vi "Connect Websockets.vi"(6 "timeout (100ms)":i32=100, 7 "path (/)":string="/", 8 "error in (no error)":errorcluster, 10 "remote port (80)":u16=80, 11 "address (localhost)":string="localhost") -> (0 "error out":errorcluster, 3 "Websockets":refnum<class "Connection.WS.lvclass">)   [LabVIEW 2013, in "MQTT_Websockets.lvlib" / "WebsocketsConnection.lvclass"]
uses:
  WebsocketsConnection.lvclass
  <vilib>/LabVIEW Open Source Project/Connection/Connection.Websockets/Connection.WS.lvclass
  <vilib>/LabVIEW Open Source Project/Connection/Connection/Connection.lvclass
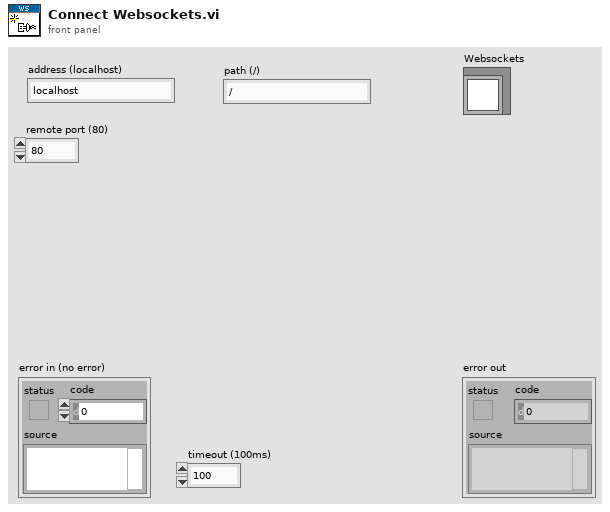
[diagram p1: front panel]
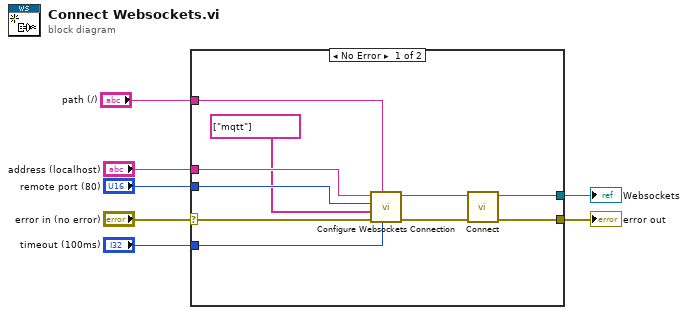
[diagram p0: block diagram]
diagram:
  n1 = case shown="No Error" "error in (no error)" {
    selector: "error in (no error)" -> [w11 w18]
    tunnel: [w16 w18] -> w6
    tunnel: [w17 _] -> w2
    tunnel: "address (localhost)" -> [w15 _]
    tunnel: "remote port (80)" -> [w14 _]
    tunnel: "timeout (100ms)" -> [w10 _]
    tunnel: "path (/)" -> [w8 _]
    frame No Error {
      n2 = call <vilib>:"Configure Websockets Connection.vi"("timeout (5000ms)"=w10, "path (/)"=w8, "error in (no error)"=w11, "subProtocols"=string[] ["mqtt"], "remote port (80)"=w14, "address (localhost)"=w15) -> ("error out"=w12:errorcluster, "Connection.Websockets"=w13:refnum<class "Connection.WS.lvclass">)  [unwired: 4 in]
      n3 = call <vilib>:"Connect.vi"("error in (no error)"=w12, "Connection in"=w13) -> ("error out"=w16:errorcluster, "Connection out"=w17:refnum<class "Connection.WS.lvclass">)  [unwired: 8 in]
    }
    frame Error {
    }
  }
  "error out" <- w6
  "Websockets" <- w2
